vi "battery normalizer.vi"(1 "input":dbl) -> (0 "output variable":dbl)   [LabVIEW 2011]
uses:
  fg_typedef.ctl
panel:
  # "use the current battery voltage to increase the shooter speed to compensate for lower battery"
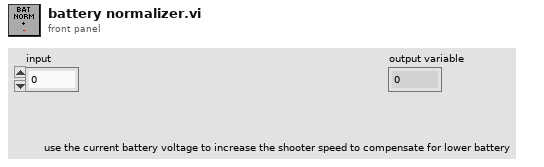
[diagram p1: front panel]
types:
  T1 = typedef "fg_typedef.ctl" = enum16{"Get", "Set"}
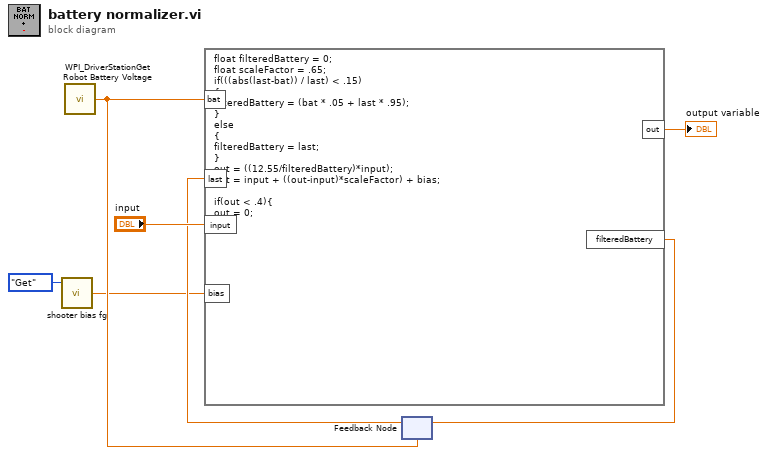
[diagram p0: block diagram]
diagram:
  n1 = call "shooter bias fg.vi"("Menu"=fg_typedef."Get") -> ("output"=w1:dbl)  [unwired: 2 in]
  n2 = call <vilib>:"WPI_DriverStationGet Robot Battery Voltage.vi"() -> ("robot battery voltage"=w3:dbl)  [unwired: 14 in, 1 out]
  n3 = feedback #1(w3) -> (w4:dbl)
  n4 = formula code="float filteredBattery = 0;\nfloat scaleFactor = .65;\nif(((abs(last-bat)) / last) < .15)\n{\nfilteredBattery = (bat * .05 + last * .95);\n}\nelse\n{\nfilteredBattery = last;\n}\nout = ((12.55/filteredBattery)*input);\nout = input + ((out-input)*scaleFactor) + bias;\n\nif(out < .4){\nout = 0;\n}"("bat"=w3, "last"=w4, "input"="input", "bias"=w1) -> ("out"=→"output variable":dbl, "filteredBattery"=w5:dbl)
  n5 = feedback-in #1(w5) -> ()
